vi "arm shoot.vi"(9 "Joystick":dbl) -> (1 "Output":dbl)   [LabVIEW 2012]
uses:
  <vilib>/addons/control/pid/pid.llb/PID (DBL).vi
  <vilib>/addons/control/pid/NI_PID_pid.lvlib
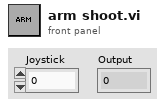
[diagram p1: front panel]
types:
  T1 = typedef "WPI_EncoderDevRef.ctl" = cluster{"DevStatus":errorcluster, "EncoderIndex":T2, "CounterIndex":T3, "DistancePerCount":dbl, "Decoding Type":T4}
  T2 = typedef "FPGA_EncoderIdx.ctl" = enum8{"Enc 0", "Enc 1", "Enc 2", "Enc 3", "Invalid"}
  T3 = typedef "FPGA_CounterCtrSystemIndex.ctl" = enum8{"Ctr 0", "Ctr 1", "Ctr 2", "Ctr 3", "Ctr 4", "Ctr 5", "Ctr 6", "Ctr 7", "Invalid"}
  T4 = typedef "WPI_EncoderType.ctl" = enum16{"1x", "2x", "4x"}
  T5 = cluster{"proportional gain (Kc)":dbl, "integral time (Ti, min)":dbl, "derivative time (Td, min)":dbl}
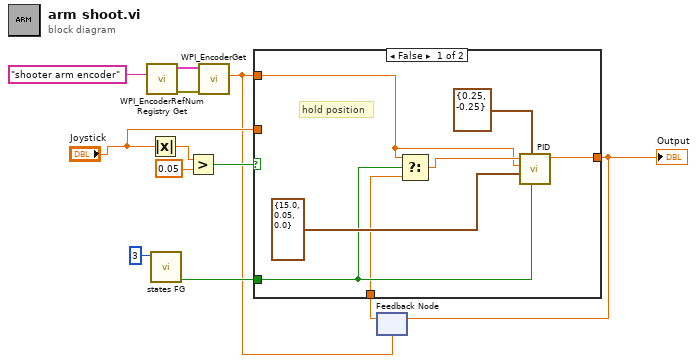
[diagram p0: block diagram]
diagram:
  n1 = call <vilib>:"WPI_EncoderRefNum Registry Get.vi"("refnum name"="shooter arm encoder") -> ("error out"=w10:errorcluster, "EncoderDevRef"=w11:T1)  [unwired: 9 in]
  n2 = Absolute Value(x="Joystick") -> (abs(x)=w5:dbl)
  n3 = call "states FG.vi"("Loop ID"=3) -> ("first call?"=w8:bool)  [unwired: 7 in, 3 out]
  n4 = Greater?(x=w5, y=0.05) -> (0:w4:bool)
  n5 = call <vilib>:"WPI_EncoderGet.vi"("error in (no error)"=w10, "EncoderDevRef"=w11) -> ("Distance"=w3:dbl)  [unwired: 4 in, 5 out]
  n6 = feedback #1(w3) -> (w2:dbl)
  n7 = case shown="False" w4 {
    tunnel: w3 -> [w14 _]
    tunnel: [w17 w20] -> w1
    tunnel: w8 -> [w16 _]
    tunnel: "Joystick" -> [_ w20]
    tunnel: w2 -> [w13 _]
    frame False {
      # "hold position"
      n8 = Select(t=w14, s=w16, f=w13) -> (s? t:f=w15:dbl)
      n9 = call-poly <vilib>:"PID.vi"("reinitialize? (F)"=w16, "output range"=cluster{"output high":dbl, "output low":dbl} {"output high"=0.25, "output low"=-0.25}, "PID gains"=T5 {"proportional gain (Kc)"=15.0, "integral time (Ti, min)"=0.05, "derivative time (Td, min)"=0.0}, "process variable"=w14, "setpoint"=w15) -> ("output"=w17:dbl)  [unwired: 5 in, 1 out]
    }
    frame True {
      # "driver control"
    }
  }
  "Output" <- w1
  n10 = feedback-in #1(w1) -> ()
